vi "Labview python test.vi"() -> ()   [LabVIEW 2022 SP3]
panel:
  out "error out 2":errorcluster
  in  "error in (no error)":errorcluster
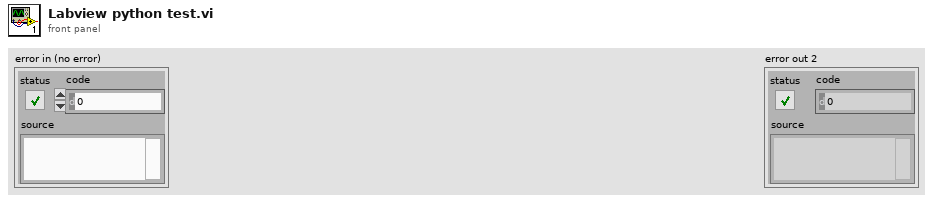
[diagram p1: front panel]
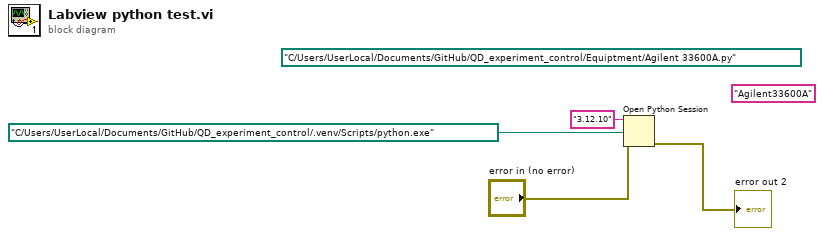
[diagram p0: block diagram]
diagram:
  (unwired) "Agilent33600A" ("function name")
  (unwired) path "C:/Users/UserLocal/Documents/GitHub/QD_experiment_control/Equiptment/Agilent 33600A.py" ("module path")
  n1 = Open Python Session(python version="3.12.10" ("Python version"), python path=path "C:/Users/UserLocal/Documents/GitHub/QD_experiment_control/.venv/Scripts/python.exe" ("Python path"), 3:"error in (no error)") -> (error out=→"error out 2":errorcluster)  [unwired: 1 out]
